vi "Build digital output.vi"(8 "error in":errorcluster, 10 "Data in":T1, 11 "Run info":T4) -> (0 "error out":errorcluster, 1 "motor cmd":u32[](array[numeric]), 2 "Data out":T1, 3 "Run info out":T4)   [LabVIEW 2012]
uses:
  Run info.ctl
  Data.ctl
  Treatment.ctl
  Treatment type.ctl
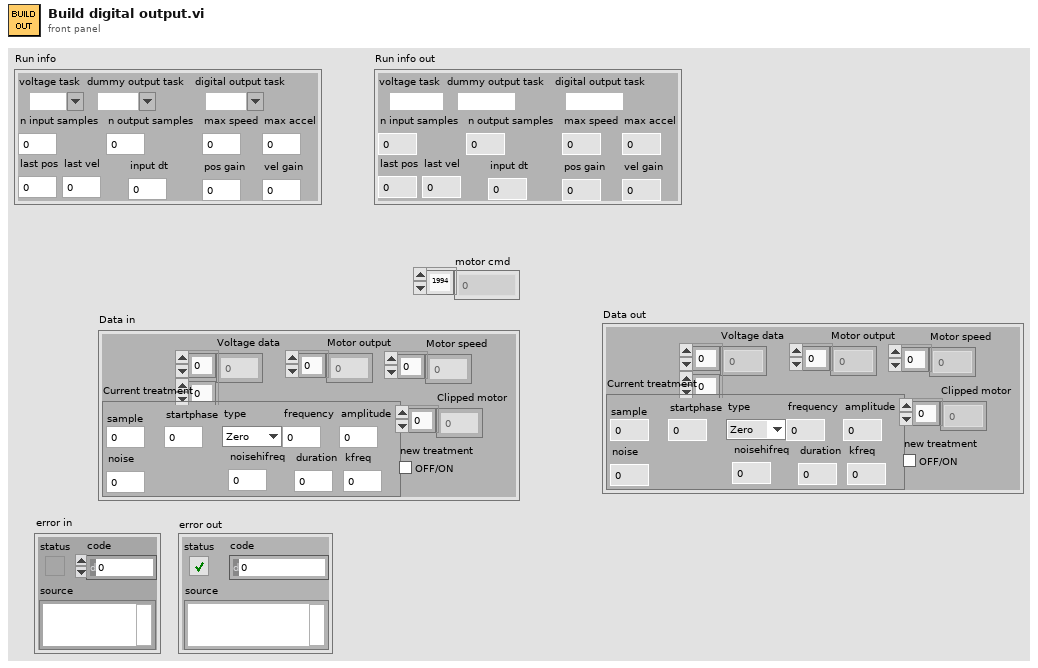
[diagram p1: front panel]
types:
  T1 = typedef "Data.ctl" = cluster{"Voltage data":dbl[][], "Motor output":dbl[], "Current treatment":T2, "Motor speed":dbl[], "Clipped motor":dbl[], "new treatment":bool}
  T2 = typedef "Treatment.ctl" = cluster{"sample":dbl, "startphase":dbl, "type":T3, "frequency":dbl, "amplitude":dbl, "noise":dbl, "duration":dbl, "kfreq":dbl, "noisehifreq":dbl}
  T3 = typedef "Treatment type.ctl" = enum16{"Zero", "Sine", "Frequency sweep"}
  T4 = typedef "Run info.ctl" = cluster{"voltage task":refnum<k21>, "dummy output task":refnum<k21>, "digital output task":refnum<k21>, "n input samples":i32, "n output samples":i32, "max speed":dbl, "max accel":dbl, "last pos":dbl, "last vel":dbl, "pos gain":dbl, "vel gain":dbl, "input dt":dbl}
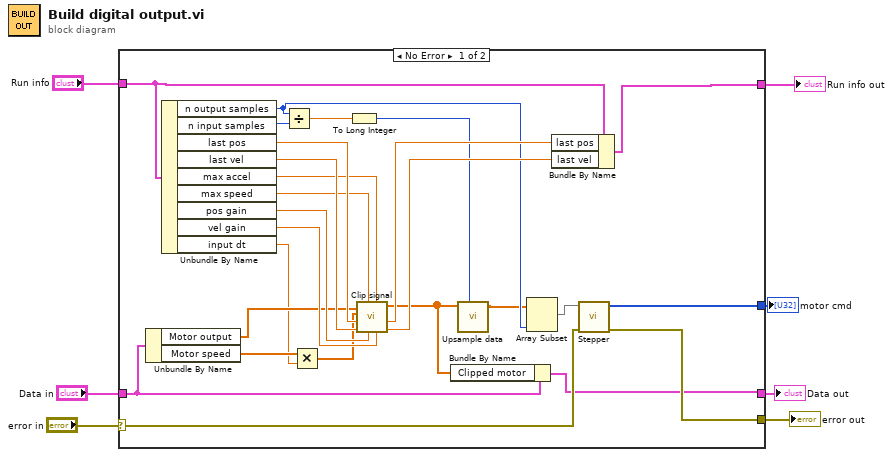
[diagram p0: block diagram]
diagram:
  n1 = case shown="No Error" "error in" {
    selector: "error in" -> [w23 w35]
    tunnel: "Run info" -> [w27 w36]
    tunnel: [w22 w35] -> w5
    tunnel: [w24 w36] -> w4
    tunnel: "Data in" -> [w12 w34]
    tunnel: [w21 _] -> w2
    tunnel: [w11 w34] -> w1
    frame No Error {
      n2 = Unbundle By Name(w12) -> ("Motor output"=w19:dbl[], "Motor speed"=w10:dbl[])
      n3 = Unbundle By Name(w27) -> ("n output samples"=w18:i32, "n input samples"=w20:i32, "last pos"=w33:dbl, "last vel"=w32:dbl, "max accel"=w30:dbl, "max speed"=w31:dbl, "pos gain"=w29:dbl, "vel gain"=w28:dbl, "input dt"=w9:dbl)
      n4 = Divide(x=w18, y=w20) -> (x/y=w16:dbl)
      n5 = Multiply(x=w10, y=w9) -> (x*y=w8:dbl[])
      n6 = To Long Integer(number=w16) -> (32bit integer=w15:i32)
      n7 = call "Clip signal.vi"("vel gain"=w28, "max accel"=w30, "pos gain"=w29, "max speed"=w31, "init vel"=w32, "init pos"=w33, "V"=w8, "Y"=w19) -> ("final vel"=w25:dbl, "final pos"=w26:dbl, "Clipped Y"=w13:dbl[])  [unwired: 1 in]
      n8 = Bundle By Name(cluster=w12, "Clipped motor"=w13) -> (w11:T1)
      n9 = call "Upsample data.vi"("factor"=w15, "data"=w13) -> ("upsampled data"=w14:dbl[])  [unwired: 9 in]
      n10 = Array Subset(array=w14, length=w18) -> (w17:dbl[])  [unwired: 1 in]
      n11 = Bundle By Name(cluster=w27, "last pos"=w26, "last vel"=w25) -> (w24:T4)
      n12 = call "Stepper.vi"("error in"=w23, "position"=w17) -> ("error out"=w22:errorcluster, "motor cmd"=w21:u32[])  [unwired: 8 in]
    }
    frame Error {
    }
  }
  "Run info out" <- w4
  "error out" <- w5
  "motor cmd" <- w2
  "Data out" <- w1
